vi "Matrix left divisionMV.vi"(2 "A":dbl[](array[numeric]), 3 "number of iterations":i32=2, 4 "B":dbl[][](array[numeric]), 5 "SVD relative tolerance":dbl) -> (0 "error":i32, 1 "B\\A":dbl[](array[numeric]))   [LabVIEW 2018, in "NI_Gmath.lvlib"]
doc: "Left division operator. B\\A solves the equation B*X=A. When used with two polynomials, \\ is overloaded to produce a transfer function whose numerator is the right-hand operand. When used with two dynamic systems, a new system is created whose state matrix is the appended states of the two systems and whose output matrix is that of the \"numerator\" system. (For systems in transfer- function format, the new system is obtained by multiplying the \"numerator\" system by the reciprocal of the \"denominator\" system.) For matrix division, there are no specific conditions on the dimensions of A and B but the condition of B affects the accuracy of the matrix quotient obtained. An error message appears if B is singular. If B is square and nonsingular, B\\A returns a matrix X with the same dimensions as A. An LU (Gaussian) decomposition, rather than a direct inverse, is used. If the condition estimate of B is less than the machine epsilon, a warning message appears. If B is non-square, X is the least-squares solution to B*X=A and has row dimension equal to the number of columns of B and column dimension equal to the number of columns of A. This operation uses a QR decomposition to implicitly compute the rank of B; the solution X will have no more nonzero components in each column than this rank value."
uses:
  NI_Gmath.lvlib
  A x Vector.vi
  Real SVD Decomposition.vi
  NI_AALBase.lvlib
  NI_AALPro.lvlib
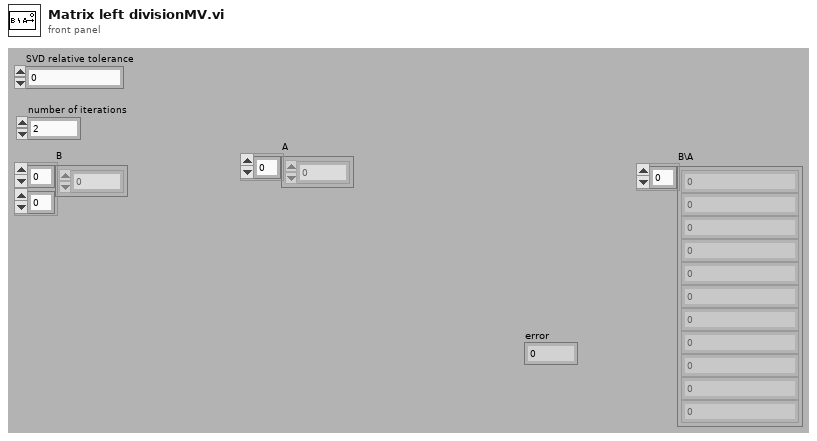
[diagram p1: front panel]
types:
  T1 = typedef "NI_Matrix.lvlib/RealMatrix.ctl" = dbl[][]
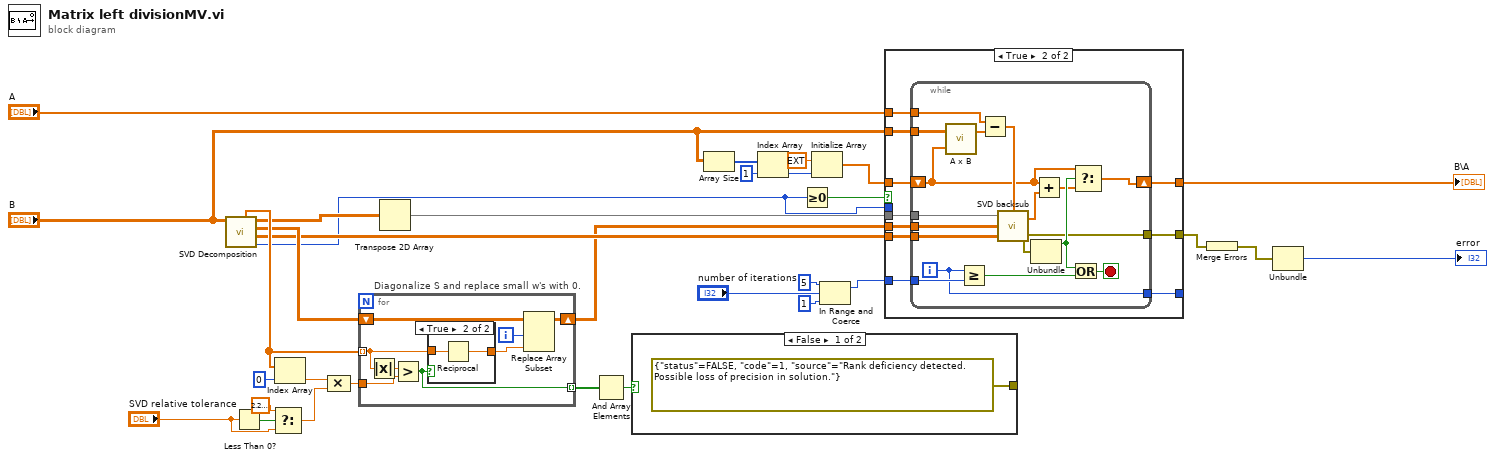
[diagram p0: block diagram]
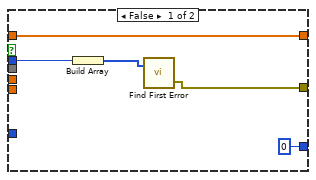
[diagram p2: hidden frame]
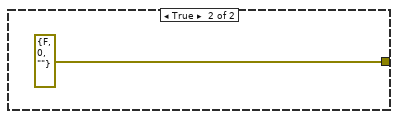
[diagram p3: hidden frame]
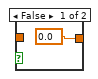
[diagram p4: hidden frame]
diagram:
  # "Diagonalize S and replace small w's with 0."
  n1 = call-poly "SVD Decomposition.vi"("A"="B") -> ("error"=w4:i32, "Matrix V"=w15:T1, "Matrix S"=w16:T1, "Matrix U"=w23:T1, "Vector S"=w24:dbl[])  [unwired: 6 in]
  n2 = Less Than 0?(x="SVD relative tolerance") -> (x < 0?=w22:bool)
  n3 = Select(t=2.220446049250313e-16, s=w22, f="SVD relative tolerance") -> (s? t:f=w20:dbl)
  n4 = Index Array(array=w24, index=0) -> (element=w26:dbl)
  n5 = Compound Arithmetic op=MULTIPLY(w26, w20) -> (w27:dbl)
  n6 = for {
    tunnel: w24 -> [w36] mode=indexing
    shift-right: [w39] -> w14
    shift-left: w16 -> [w38]
    tunnel: w27 -> [w34]
    tunnel: [w33] -> w19 mode=indexing
    i -> [w40]
    n7 = Absolute Value(x=w36) -> (abs(x)=w35:dbl)
    n8 = Greater?(x=w35, y=w34) -> (0:w33:bool)
    n9 = case shown="True" w33 {
      tunnel: w36 -> [_ w43]
      tunnel: [0.0 w42] -> w37
      frame False {
      }
      frame True {
        n10 = Reciprocal(x=w43) -> (1/x=w42:dbl)
      }
    }
    n11 = Replace Array Subset(array=w38, new element=w37, index (row)=w40, index (col)=w40) -> (w39:T1)
  }
  n12 = Transpose 2D Array(2D array=w23) -> (transposed array=w13:T1)
  n13 = And Array Elements(Boolean array=w19) -> (logical AND=w18:bool)
  n14 = case shown="False" w18 {
    tunnel: [errorcluster {"status"=FALSE, "code"=1, "source"="Rank deficiency detected.  Possible loss of precision in solution."} ("error out") errorcluster {"status"=FALSE, "code"=0, "source"=""} ("error out")] -> _
    frame False {
    }
    frame True {
    }
  }
  n15 = Array Size(array="B") -> (size(s)=w11:i32[])
  n16 = Index Array(array=w11, index=1) -> (element=w3:i32)
  n17 = Greater Or Equal To 0?(x=w4) -> (x >= 0?=w5:bool)
  n18 = Initialize Array(ext 0.0 ("element"), w3) -> (w28:ext[])
  n19 = In Range and Coerce(upper limit=5, x="number of iterations", lower limit=1) -> (coerced(x)=w6:i32)  [unwired: 1 out]
  n20 = case shown="True" w5 {
    tunnel: "B" -> [_ w60]
    tunnel: [w50 w59] -> w29
    tunnel: w28 -> [w50 w58]
    tunnel: "A" -> [_ w57]
    tunnel: w15 -> [_ w56]
    tunnel: w14 -> [_ w55]
    tunnel: w13 -> [_ w54]
    tunnel: w6 -> [_ w53]
    tunnel: [w47 w52] -> w12
    tunnel: [0 w51] -> _
    tunnel: w4 -> [w49 _]
    frame False {
      n21 = Build Array(w49) -> (w48:i32[])
      n22 = call "Find First Error.vi"("error codes"=w48) -> ("error out"=w47:errorcluster)  [unwired: 3 in, 1 out]
    }
    frame True {
      n23 = while {
        shift-right: [w66] -> w59
        shift-left: w58 -> [w65]
        tunnel: w60 -> [w77]
        tunnel: w57 -> [w63]
        tunnel: w54 -> [w75]
        tunnel: w55 -> [w74]
        tunnel: w56 -> [w73]
        tunnel: w53 -> [w71]
        tunnel: [w64] -> w52
        tunnel: [w61] -> w51
        i -> [w61]
        stop <- w69 stop-if-true
        n24 = call-poly "A x B.vi"("Vector"=w65, "A"=w77) -> ("A x Vector"=w62:dbl[])  [unwired: 1 out]
        n25 = Greater Or Equal?(x=w61, y=w71) -> (x >= y?=w70:bool)
        n26 = Subtract(x=w63, y=w62) -> (x-y=w72:dbl[])
        n27 = call "SVD backsub.vi"("A"=w72, "V"=w73, "1/S"=w74, "U^T"=w75) -> ("error out"=w64:errorcluster, "solution"=w76:dbl[])
        n28 = Unbundle(w64) -> ("status"=w68:bool)  [unwired: 2 out]
        n29 = Add(x=w65, y=w76) -> (x+y=w67:ext[])
        n30 = Or(x=w68, y=w70) -> (x .or. y?=w69:bool)
        n31 = Select(t=w65, s=w68, f=w67) -> (s? t:f=w66:ext[])
      }
    }
  }
  "B\\A" <- w29
  n32 = Merge Errors(w12) -> (w1:errorcluster)
  n33 = Unbundle(w1) -> ("code"=→"error":i32)  [unwired: 2 out]
